vi "4PTSCalibCheck.vi"(9 "IdealPointIn(A)":cluster{"PTX1":dbl, "PTY1":dbl}, 10 "InputRobot(B)":T1, 11 "InputIdeal(A)":T1) -> (3 "RobotOut(B )":cluster{"RX":dbl, "RY":dbl})   [LabVIEW 2019]
uses:
  <vilib>/Analysis/baseanly.llb/Matrix Type of Inverse Matrix.ctl
  <vilib>/Analysis/baseanly.llb/Real A x B.vi
  <vilib>/Analysis/baseanly.llb/A x Vector.vi
  <vilib>/Analysis/baseanly.llb/Real Inverse Matrix.vi
  <vilib>/Analysis/NI_AALBase.lvlib
panel:
  out "A x Vector":dbl[](array[numeric]) format="%.2f"
  out "appended array":dbl[][](array[numeric])
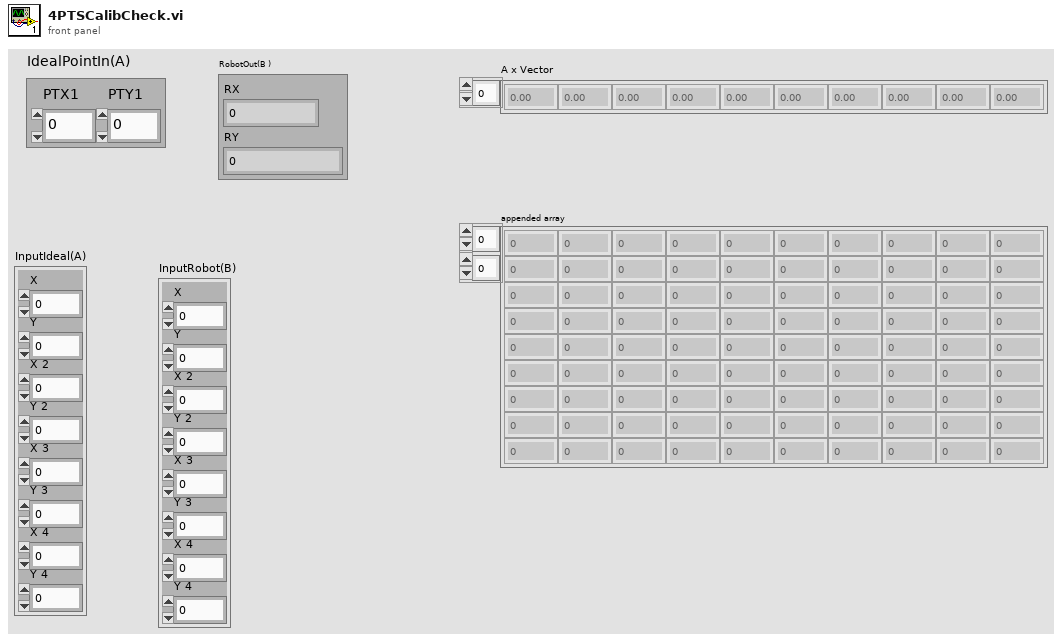
[diagram p1: front panel]
types:
  T1 = cluster{"X":dbl, "Y":dbl, "X 2":dbl, "Y 2":dbl, "X 3":dbl, "Y 3":dbl, "X 4":dbl, "Y 4":dbl}
  T2 = typedef "NI_AALBase.lvlib/Matrix Type of Inverse Matrix.ctl" = enum32{"General", "Positive Definite", "Lower Triangular", "Upper Triangular"}
  T3 = typedef "NI_Matrix.lvlib/RealMatrix.ctl" = dbl[][]
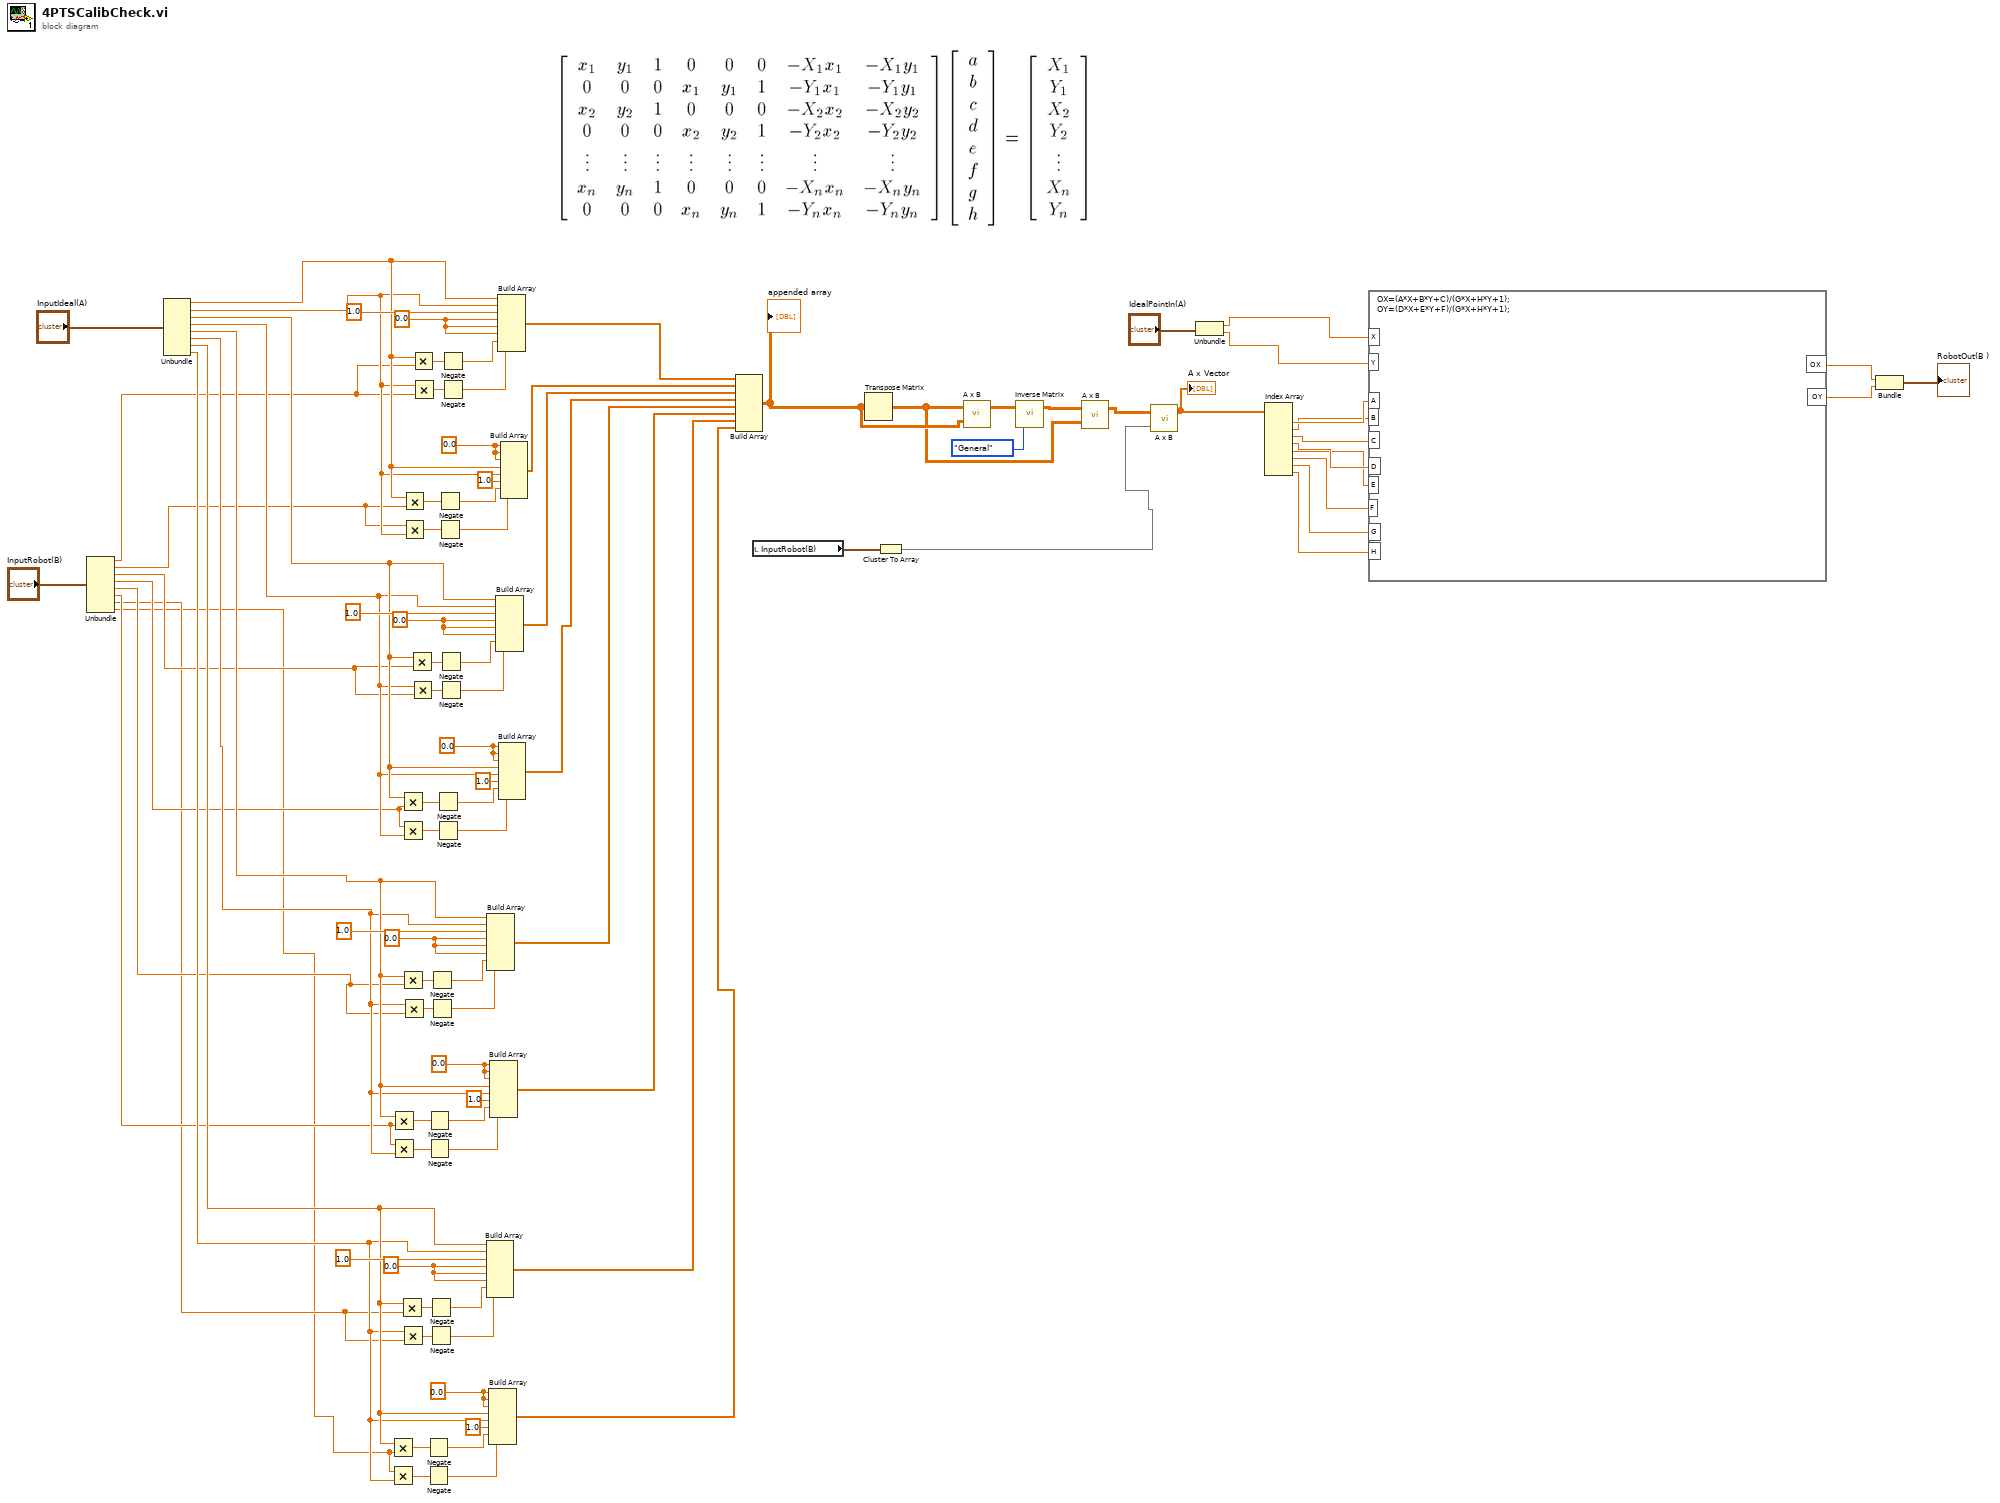
[diagram p0: block diagram]
diagram:
  w56 = 0.0 ("element")
  w51 = 0.0 ("element")
  w67 = 0.0 ("element")
  w72 = 0.0 ("element")
  w80 = 0.0 ("element")
  w75 = 0.0 ("element")
  w91 = 0.0 ("element")
  w96 = 0.0 ("element")
  n1 = Unbundle("InputRobot(B)") -> ("X"=w16:dbl, "Y"=w15:dbl, "X 2"=w14:dbl, "Y 2"=w13:dbl, "X 3"=w12:dbl, "Y 3"=w11:dbl, "X 4"=w10:dbl, "Y 4"=w9:dbl)
  n2 = Unbundle("InputIdeal(A)") -> ("X"=w25:dbl, "Y"=w24:dbl, "X 2"=w23:dbl, "Y 2"=w22:dbl, "X 3"=w21:dbl, "Y 3"=w20:dbl, "X 4"=w19:dbl, "Y 4"=w18:dbl)
  n3 = Multiply(x=w19, y=w9) -> (x*y=w58:dbl)
  n4 = Multiply(x=w9, y=w18) -> (x*y=w60:dbl)
  n5 = Multiply(x=w21, y=w11) -> (x*y=w65:dbl)
  n6 = Multiply(x=w11, y=w20) -> (x*y=w63:dbl)
  n7 = Multiply(x=w19, y=w10) -> (x*y=w52:dbl)
  n8 = Multiply(x=w23, y=w13) -> (x*y=w82:dbl)
  n9 = Multiply(x=w13, y=w22) -> (x*y=w84:dbl)
  n10 = Multiply(x=w21, y=w12) -> (x*y=w71:dbl)
  n11 = Multiply(x=w18, y=w10) -> (x*y=w54:dbl)
  n12 = Multiply(x=w20, y=w12) -> (x*y=w69:dbl)
  n13 = Multiply(x=w25, y=w15) -> (x*y=w89:dbl)
  n14 = Multiply(x=w15, y=w24) -> (x*y=w87:dbl)
  n15 = Multiply(x=w23, y=w14) -> (x*y=w76:dbl)
  n16 = Multiply(x=w22, y=w14) -> (x*y=w78:dbl)
  n17 = Multiply(x=w25, y=w16) -> (x*y=w95:dbl)
  n18 = Multiply(x=w24, y=w16) -> (x*y=w93:dbl)
  n19 = Negate(x=w58) -> (-x=w59:dbl)
  n20 = Negate(x=w60) -> (-x=w61:dbl)
  n21 = Negate(x=w65) -> (-x=w64:dbl)
  n22 = Negate(x=w63) -> (-x=w62:dbl)
  n23 = Negate(x=w52) -> (-x=w53:dbl)
  n24 = Negate(x=w54) -> (-x=w55:dbl)
  n25 = Negate(x=w71) -> (-x=w70:dbl)
  n26 = Negate(x=w69) -> (-x=w68:dbl)
  n27 = Negate(x=w82) -> (-x=w83:dbl)
  n28 = Negate(x=w84) -> (-x=w85:dbl)
  n29 = Negate(x=w89) -> (-x=w88:dbl)
  n30 = Negate(x=w87) -> (-x=w86:dbl)
  n31 = Negate(x=w76) -> (-x=w77:dbl)
  n32 = Negate(x=w78) -> (-x=w79:dbl)
  n33 = Negate(x=w95) -> (-x=w94:dbl)
  n34 = Negate(x=w93) -> (-x=w92:dbl)
  n35 = Build Array(w19, w18, 1.0 ("element"), w51, w51, w51, w53, w55) -> (w43:dbl[])
  n36 = Build Array(w21, w20, 1.0 ("element"), w72, w72, w72, w70, w68) -> (w45:dbl[])
  n37 = Build Array(w56, w56, w56, w19, w18, 1.0 ("element"), w59, w61) -> (w42:dbl[])
  n38 = Build Array(w67, w67, w67, w21, w20, 1.0 ("element"), w64, w62) -> (w44:dbl[])
  n39 = Build Array(w23, w22, 1.0 ("element"), w75, w75, w75, w77, w79) -> (w47:dbl[])
  n40 = Build Array(w25, w24, 1.0 ("element"), w96, w96, w96, w94, w92) -> (w49:dbl[])
  n41 = Build Array(w80, w80, w80, w23, w22, 1.0 ("element"), w83, w85) -> (w46:dbl[])
  n42 = Build Array(w91, w91, w91, w25, w24, 1.0 ("element"), w88, w86) -> (w48:dbl[])
  n43 = Build Array(w49, w48, w47, w46, w45, w44, w43, w42) -> (w41:dbl[][])
  "appended array" <- w41
  n44 = local read "InputRobot(B)"() -> (w8:T1)
  n45 = Transpose Matrix(1:w41) -> (0:w39:dbl[][])
  n46 = Cluster To Array(cluster=w8) -> (array=w7:dbl[])
  n47 = call-poly <vilib>:"A x B.vi"("B"=w41, "A"=w39) -> ("A x B"=w40:T3)  [unwired: 1 out]
  n48 = call-poly <vilib>:"Inverse Matrix.vi"("matrix type"=Matrix_Type_of_Inverse_Matrix."General", "Input Matrix"=w40) -> ("Inverse Matrix"=w38:T3)  [unwired: 1 out]
  n49 = call-poly <vilib>:"A x B.vi"("B"=w39, "A"=w38) -> ("A x B"=w37:T3)  [unwired: 1 out]
  n50 = call-poly <vilib>:"A x B.vi"("Vector"=w7, "A"=w37) -> ("A x Vector"=w35:dbl[])  [unwired: 1 out]
  "A x Vector" <- w35
  n51 = Unbundle("IdealPointIn(A)") -> ("PTX1"=w2:dbl, "PTY1"=w1:dbl)
  n52 = Index Array(array=w35) -> (element #1=w34:dbl, element #2=w33:dbl, element #3=w32:dbl, element #4=w31:dbl, element #5=w30:dbl, element #6=w29:dbl, element #7=w28:dbl, element #8=w27:dbl)  [unwired: 8 in]
  n53 = formula code="OX=(A*X+B*Y+C)/(G*X+H*Y+1);\nOY=(D*X+E*Y+F)/(G*X+H*Y+1);"("X"=w2, "Y"=w1, "A"=w34, "B"=w33, "C"=w32, "D"=w31, "E"=w30, "F"=w29, "G"=w28, "H"=w27) -> ("OY"=w5:dbl, "OX"=w6:dbl)
  n54 = Bundle("OX"=w6, "OY"=w5) -> (→"RobotOut(B )":cluster{"OX":dbl, "OY":dbl})  [unwired: 1 in]
